vi "GetParam.vi"(8 "error in (no error)":errorcluster caption="entrée d'erreur (pas d'erreur)", 11 "scale.lvclass":refnum<class "scale.lvclass">) -> (0 "error out":errorcluster caption="sortie d'erreur", 2 "scale":T1={"axis"=0, "with_mean"=TRUE, "with_std"=TRUE, "copy"=TRUE}, 3 "scale.lvclass":refnum<class "scale.lvclass">)   [LabVIEW 2020, in "scale.lvclass"]
doc: "Get Parameters"
uses:
  scale.lvclass
  scale.lvclass/scale.ctl
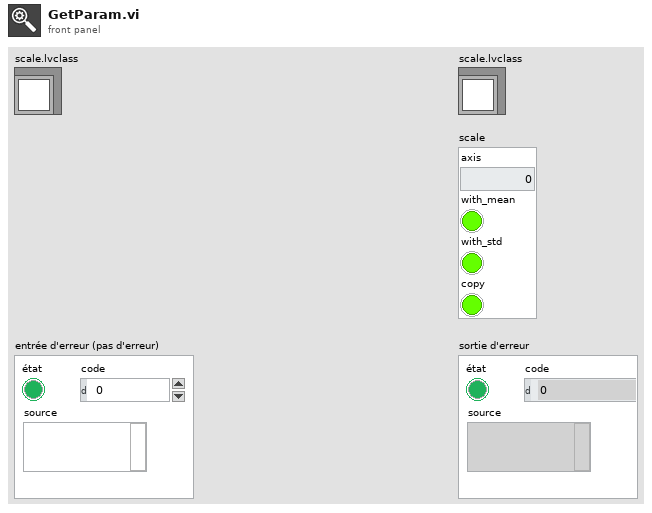
[diagram p1: front panel]
types:
  T1 = cluster{"axis":i32, "with_mean":bool, "with_std":bool, "copy":bool}
  T2 = cluster{"axis":u8, "with_mean":bool, "with_std":bool, "copy":bool}
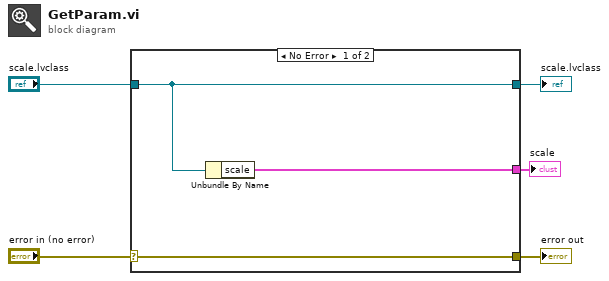
[diagram p0: block diagram]
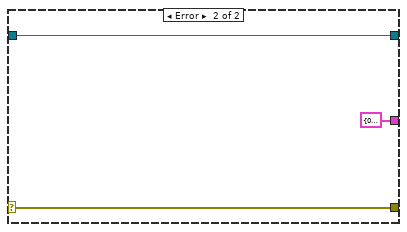
[diagram p2: hidden frame]
diagram:
  n1 = case shown="No Error" "error in (no error)" {
    selector: "error in (no error)" -> [w8 w10]
    tunnel: [w8 w10] -> w4
    tunnel: [w7 w11] -> w2
    tunnel: "scale.lvclass" -> [w7 w11]
    tunnel: [w6 T2 {"axis"=0, "with_mean"=FALSE, "with_std"=FALSE, "copy"=FALSE} ("scale")] -> w1
    frame No Error {
      n2 = Unbundle By Name(w7) -> ("scale"=w6:T1)
    }
    frame Error {
    }
  }
  "error out" <- w4
  "scale.lvclass" <- w2
  "scale" <- w1
